vi "Quaternion_Plus.vi"(9 "Other Quaternion":T1={"R"=1.0, "V"=[0.0, 0.0, 0.0]}, 11 "Quaternion":T1={"R"=1.0, "V"=[0.0, 0.0, 0.0]}) -> (3 "Sum":T1={"R"=1.0, "V"=[0.0, 0.0, 0.0]})   [LabVIEW 2019, in "Trajectory_Library.lvlib"]
doc: "Sum with another quaternion.\n\nParameters:\n - Quaternion - The quaternion data cluster\n - Other Quaternion - The other quaternion data cluster\n\nReturns:\n - Sum - The quaternion summation."
uses:
  Trajectory_Library.lvlib
  TypeDef/QUATERNION.ctl
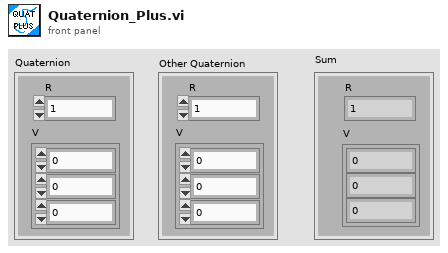
[diagram p1: front panel]
types:
  T1 = typedef "Trajectory_Library.lvlib/QUATERNION.ctl" = cluster{"R":dbl, "V":dbl[]}
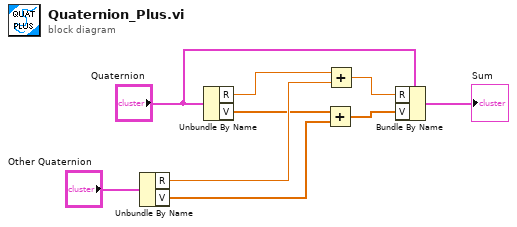
[diagram p0: block diagram]
diagram:
  n1 = Unbundle By Name("Other Quaternion") -> ("R"=w6:dbl, "V"=w5:dbl[])
  n2 = Unbundle By Name("Quaternion") -> ("R"=w4:dbl, "V"=w3:dbl[])
  n3 = Add(x=w3, y=w5) -> (x+y=w1:dbl[])
  n4 = Add(x=w4, y=w6) -> (x+y=w2:dbl)
  n5 = Bundle By Name(cluster="Quaternion", "R"=w2, "V"=w1) -> (→"Sum":T1)
